vi "FIFO Flush-variable length FIFO.vi"(8 "error in":errorcluster, 11 "FPGA VI Ref":T1) -> (0 "error out":errorcluster, 3 "FPGA VI Reference Out":T1)   [LabVIEW 2020]
uses:
  <vilib>/rvi/interface/nirviMethod/nirviMethod.xnode
  <vilib>/rvi/errors/niLvFpgaMergeErrorWithErrorCode.vi
  RIG-SPECIFIC FILES/FPGA Refs/FPGA Ref.ctl
  <vilib>/FPGAPlugInAG/Dynamic/niLvFpga_AcquireWriteRegionFifo_Dynamic.vi
  <vilib>/FPGAPlugInAG/Dynamic/niLvFpga_ReadFifo_Dynamic.vi
panel:
  in  "Manual force stop":bool
  out "Data Inter trial Time":u64[](array[numeric])
  out "Inter trial time zero":u32
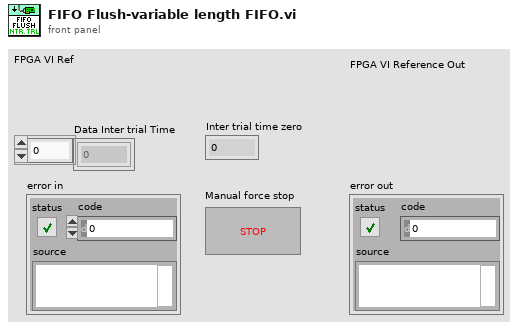
[diagram p1: front panel]
types:
  T1 = typedef "FPGA Ref.ctl" = refnum<k20>
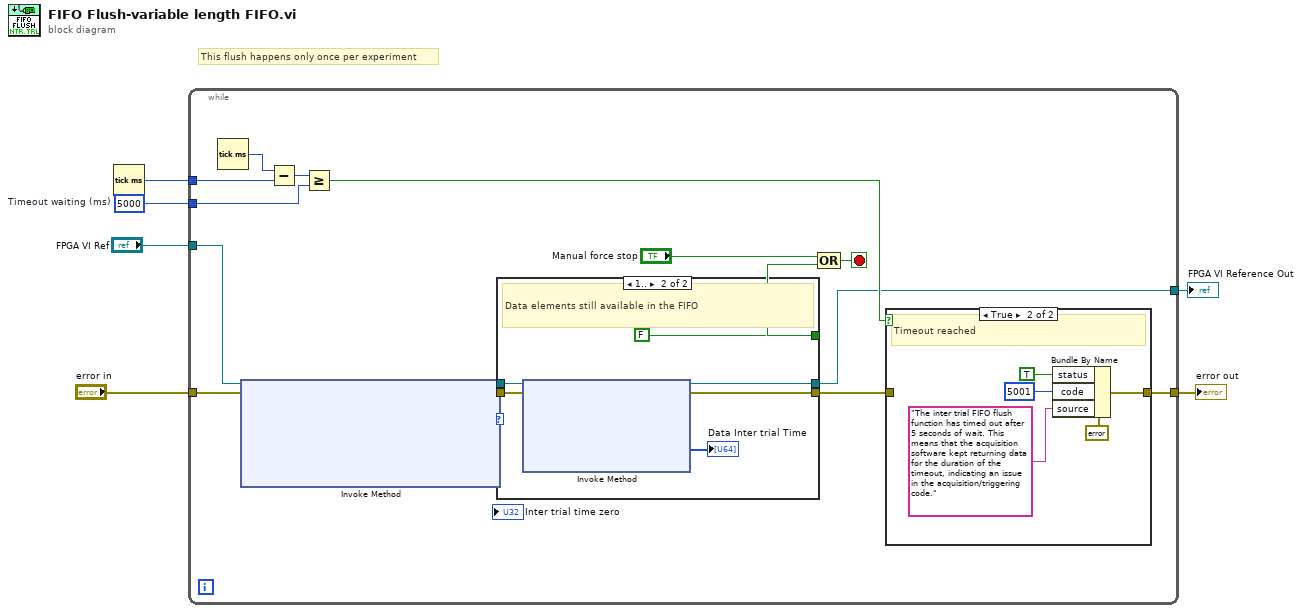
[diagram p0: block diagram]
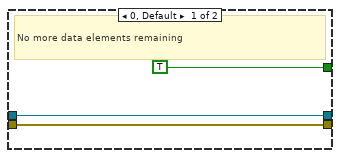
[diagram p2: hidden frame]
diagram:
  w5 = u32 5000  # Timeout waiting (ms)
  # "This flush happens only once per experiment"
  n1 = Tick Count (ms)() -> (millisecond timer value=w6:u32)
  n2 = while {
    tunnel: w6 -> [w18]
    tunnel: w5 -> [w19]
    tunnel: "FPGA VI Ref" -> [w14]
    tunnel: "error in" -> [w13]
    tunnel: [w8] -> w2
    tunnel: [w7] -> w1
    stop <- w11 stop-if-true
    n3 = Tick Count (ms)() -> (millisecond timer value=w21:u32)
    n4 = xnode "Invoke Method"("FPGA VI Reference In"=w14, "error in"=w13) -> ("FPGA VI Reference Out"=w16:T1, "error out"=w15:errorcluster)  [unwired: 2 in, 3 out]
    n5 = Subtract(x=w21, y=w18) -> (x-y=w20:u32)
    n6 = Greater Or Equal?(x=w20, y=w19) -> (x >= y?=w17:bool)
    n7 = case shown="1.." {
      selector: _ -> [_ _]
      tunnel: w15 -> [w23 w31]
      tunnel: w16 -> [w22 w30]
      tunnel: [w23 w29] -> w9
      tunnel: [TRUE FALSE] -> w10
      tunnel: [w22 w25] -> w7
      frame 0, Default {
        # "No more data elements remaining"
      }
      frame 1.. {
        # "Data elements still available in the FIFO"
        n8 = xnode "Invoke Method"("FPGA VI Reference In"=w30, "error in"=w31) -> ("FPGA VI Reference Out"=w25:T1, "error out"=w29:errorcluster, "Number of Elements"=w28:u32, "Data"=→"Data Inter trial Time":u64[])  [unwired: 1 in, 1 out]
      }
    }
    n9 = Compound Arithmetic op=OR("Manual force stop", w10) -> (w11:bool)
    n10 = case shown="True" w17 {
      tunnel: [w32 w33] -> w8
      tunnel: w9 -> [w32 _]
      frame False {
      }
      frame True {
        # "Timeout reached"
        n11 = Bundle By Name(cluster=errorcluster {"status"=TRUE, "code"=5001, "source"=""} ("error out"), "status"=TRUE, "code"=5001, "source"="The inter trial FIFO flush function has timed out after 5 seconds of wait. This means that the acquisition software kept returning data for the duration of the timeout, indicating an issue in the acquisition/triggering code." ("Error Source")) -> (w33:errorcluster)
      }
    }
  }
  "error out" <- w2
  "FPGA VI Reference Out" <- w1
